vi "FlatToRichcif_manager_QueryAllChannelsRequest.vi"(5 "OutputClusterType":T1, 11 "InputCluster":T4) -> (3 "OutputCluster":T1)   [LabVIEW 2021, in "CIF_Manager_client.lvlib"]
uses:
  CIF_Manager_client.lvlib
  cif_manager_QueryAllChannelsRequest_Flat.ctl
  cif_management_common_ChannelFilter_Flat.ctl
  cif_management_common_ChannelDirection.ctl
  cif_manager_QueryAllChannelsRequest.ctl
  cif_management_common_ChannelFilter.ctl
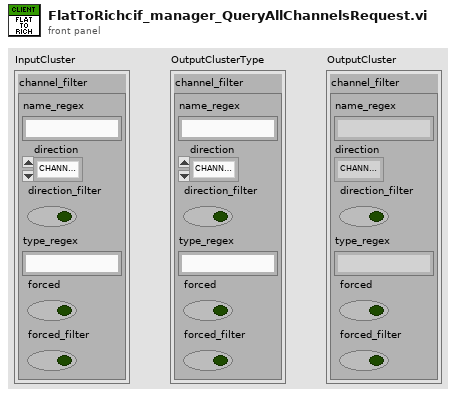
[diagram p1: front panel]
types:
  T1 = typedef "CIF_Manager_client.lvlib/cif_manager_QueryAllChannelsRequest.ctl" = cluster{"channel_filter":T2}
  T2 = typedef "CIF_Manager_client.lvlib/cif_management_common_ChannelFilter.ctl" = cluster{"name_regex":string, "direction":T3, "direction_filter":bool, "type_regex":string, "forced":bool, "forced_filter":bool}
  T3 = typedef "CIF_Manager_client.lvlib/cif_management_common_ChannelDirection.ctl" = enum32{"CHANNELDIRECTION_UNKNOWN", "CHANNELDIRECTION_PUBLISHER", "CHANNELDIRECTION_SUBSCRIBER"}
  T4 = typedef "CIF_Manager_client.lvlib/cif_manager_QueryAllChannelsRequest_Flat.ctl" = cluster{"channel_filter":T5}
  T5 = typedef "CIF_Manager_client.lvlib/cif_management_common_ChannelFilter_Flat.ctl" = cluster{"name_regex":string, "direction":T3, "direction_filter":bool, "type_regex":string, "forced":bool, "forced_filter":bool}
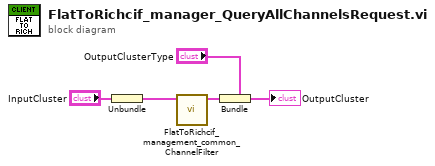
[diagram p0: block diagram]
diagram:
  n1 = Unbundle "Unbundle"("InputCluster") -> ("channel_filter"=w2:T5)
  n2 = call "FlatToRichcif_management_common_ChannelFilter.vi"("InputCluster"=w2) -> ("OutputCluster"=w1:T2)  [unwired: 10 in]
  n3 = Bundle "Bundle"(cluster="OutputClusterType", "channel_filter"=w1) -> (→"OutputCluster":T1)
